vi "analog Variables.vi"(11 "error in (no error)":errorcluster) -> (15 "error out":errorcluster)   [LabVIEW 2011]
uses:
  Variable List Common Digital.ctl
  Fixed Digital Channel Definition.ctl
  Update frequensies.ctl
  Channel catagory Enum.ctl
  <vilib>/Utility/VariantDataType/GetNumericInfo.vi
  emi Lib/Basic/0 - General/App/emi_Application Folder.vi
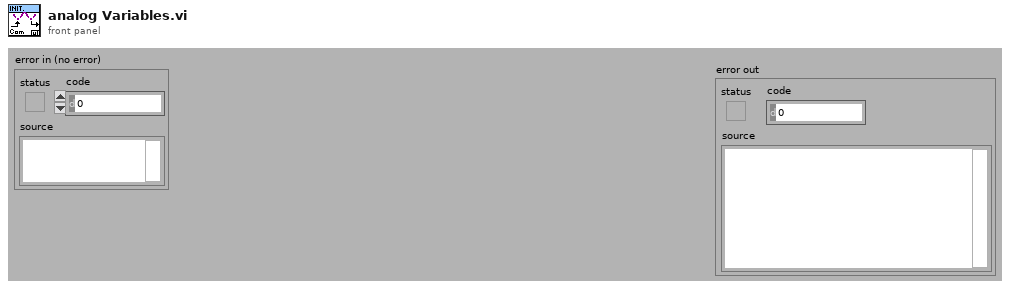
[diagram p1: front panel]
types:
  T1 = typedef "Channel catagory Enum.ctl" = enum16{"No Category", "Power", "Temperature", "Pressure"}
  T2 = typedef "Fixed Digital Channel Definition.ctl" = cluster{"ID":u16, "Name":string, "NA Text":string, "Off Text":string, "On Text":string, "Maximum upd":T3, "Comment":string, "Help file Name":string, "Help file Section ":string, "Catagory":T1, "In use":bool}
  T3 = typedef "Update frequensies.ctl" = enum16{"2 Hz", "1 Hz", "0.1 Hz"}
  T4 = typedef "Variable List Common Digital.ctl" = enum16{"PCP Connected", "PCP PC Control", "HV PSU connected", "HV PSU HV Active", "Modem Connected", "Tool Connected", "CanBus interface"}
  T5 = typedef "Fixed Analog Channel Definition.ctl" = cluster{"ID":u16, "Name":string, "Quantity":T6, "Unit":string, "Maximum upd":T3, "Comment":string, "Help file Name":string, "Help file Section ":string, "Category":T1, "User adjustable Scaling":bool, "Default Scaling":T7, "Default Unit":i32, "Classification":T8}
  T6 = typedef "Quantity enum.ctl" = enum16{"NA", "Acceleration", "Angle", "Current", "Force", "Distance", "Pressure", "Resistance", "Rotational Speed", "Speed", "Temperature", "Tension", "Torque", "Voltage", "Weight"}
  T7 = typedef "Scaling.ctl" = cluster{"Gain":dbl, "Offset":dbl}
  T8 = typedef "Channel Classification Enum.ctl" = enum16{"Basic", "Advanced", "Expert", "Unused"}
  T9 = typedef "User Setting DigitalChannel.ctl" = cluster{"Responses":cluster{"Technical Error (NA)":T10, "OFF / FALSE":T12, "ON / TRUE":T12}}
  T10 = typedef "Alarm Responce.ctl" = cluster{"Action":T11, "Alarm":bool}
  T11 = typedef "Action List.ctl" = enum16{"No Action", "Stop Motor", "Turn Off HV"}
  T12 = typedef "Alarm Responce dig.ctl" = cluster{"Action":T11, "Alarm":bool, "Exclamation":bool}
  T13 = typedef "User Setting Analog Channel Bg.ctl" = cluster{"Scaling":T7, "Limits and responces":T14, "Allow Graph selection by user":bool, "Unit":u16}
  T14 = typedef "Alarm Setup Analog.ctl" = cluster{"Technical Error(NA)":T10, "LL":T10, "L":T10, "H":T10, "HH":T10, "Limits":T15}
  T15 = typedef "Limits.ctl" = cluster{"LL":dbl, "L":dbl, "H":dbl, "HH":dbl}
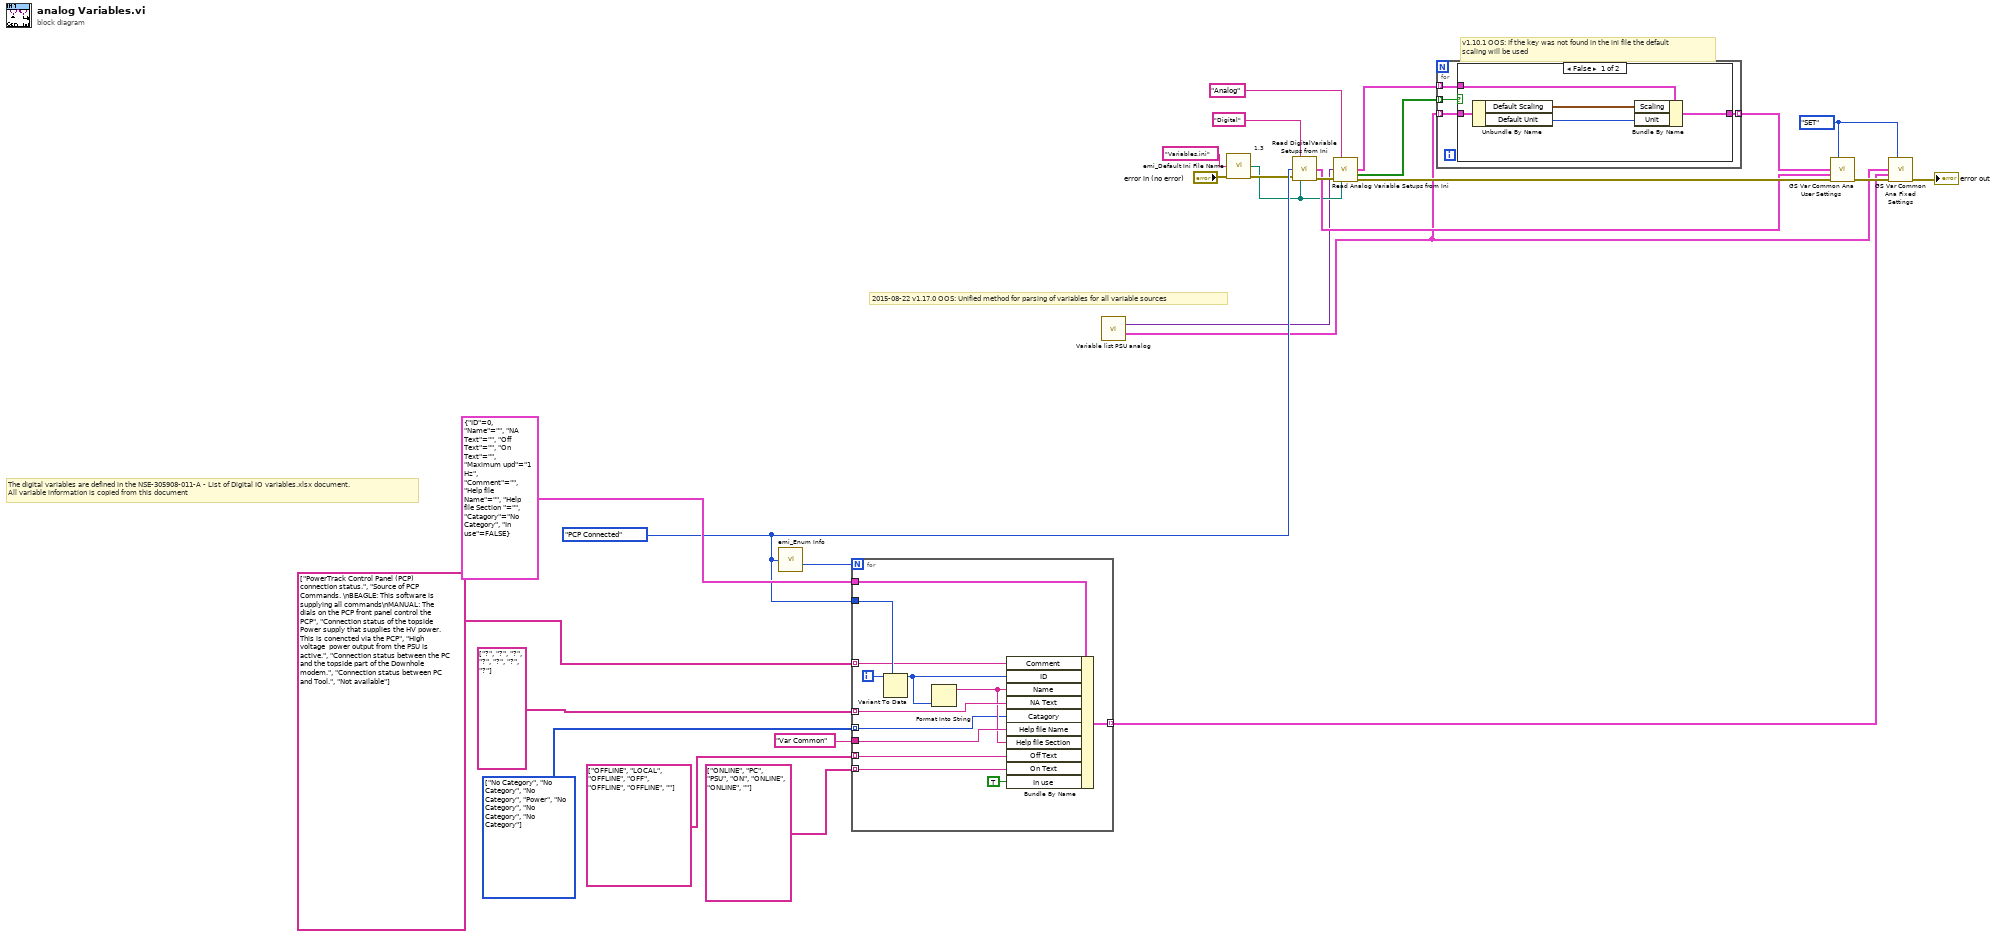
[diagram p0: block diagram]
diagram:
  w18 = T1[] [enum."No Category", enum."No Category", enum."No Category", enum."Power", enum."No Category", enum."No Category", enum."No Category"] items=["No Category", "Power", "Temperature", "Pressure"]
  w12 = Variable_List_Common_Digital."PCP Connected" ("Action")
  w24 = enum16{"GET", "SET"}."SET" ("Action(GET)")
  # "2015-08-22 v1.17.0 OOS: Unified method for parsing of variables for all variable sources"
  # "The digital variables are defined in the NSE-305908-011-A - List of Digital IO variables.xlsx document.\nAll variable information is copied from this document"
  # "v1.10.1 OOS: If the key was not found in the ini file the default\nscaling will be used"
  # "1.3"
  n1 = call "emi_Enum Info.vi"("Enum"=w12) -> ("Numb Elements"=w21:i32)  [unwired: 11 in, 3 out]
  n2 = for {
    N: w21 -> [_]
    tunnel: w12 -> [w40]
    tunnel: T2 {"ID"=0, "Name"="", "NA Text"="", "Off Text"="", "On Text"="", "Maximum upd"=enum."1 Hz", "Comment"="", "Help file Name"="", "Help file Section "="", "Catagory"=enum."No Category", "In use"=FALSE} ("Variable Defenition") -> [w37]
    tunnel: [w38] -> w15 mode=indexing
    tunnel: string[] ["?", "?", "?", "?", "?", "?", "?"] -> [w36] mode=indexing
    tunnel: w18 -> [w32] mode=indexing
    tunnel: "Var Common" -> [w34]
    tunnel: string[] ["OFFLINE", "LOCAL", "OFFLINE", "OFF", "OFFLINE", "OFFLINE", ""] -> [w31] mode=indexing
    tunnel: string[] ["ONLINE", "PC", "PSU", "ON", "ONLINE", "ONLINE", ""] -> [w30] mode=indexing
    tunnel: string[] ["PowerTrack Control Panel (PCP) connection status.", "Source of PCP Commands. \nBEAGLE: This software is supplying all commands\nMANUAL: The dials on the PCP front panel control the PCP", "Connection status of the topside Power supply that supplies the HV power. This is conencted via the PCP", "High voltage  power output from the PSU is active.", "Connection status between the PC and the topside part of the Downhole modem.", "Connection status between PC and Tool.", "Not available"] -> [w29] mode=indexing
    i -> [w35]
    n3 = Variant To Data(type=w40, Variant=w35) -> (data=w39:T4)  [unwired: 1 in, 1 out]
    n4 = Format Into String(w39) -> (resulting string=w33:string)  [unwired: 3 in, 1 out]
    n5 = Bundle By Name(cluster=w37, "Comment"=w29, "ID"=w39, "Name"=w33, "NA Text"=w36, "Catagory"=w32, "Help file Name"=w34, "Help file Section"=w33, "Off Text"=w31, "On Text"=w30, "In use"=TRUE) -> (w38:T2)
  }
  n6 = call "Variable list PSU analog.vi"() -> ("Variant"=w1:variant, "Array"=w2:T5[])  [unwired: 14 in]
  n7 = call "emi_Default Ini File Name.vi"("Name"="Variables.ini" ("name or relative path"), "error in (no error)"="error in (no error)") -> ("Path"=w6:path, "error out"=w8:errorcluster)  [unwired: 12 in]
  n8 = call "Read DigitalVariable Setups from Ini.vi"("error in (no error)"=w8, "Path"=w6, "Enum with Variable List"=w12, "Section(\"Default\")"="Digital" ("Section(\"Default\")")) -> ("error out"=w14:errorcluster, "Digitale User settigns"=w11:T9[])  [unwired: 10 in]
  n9 = call "Read Analog Variable Setups from Ini.vi"("error in (no error)"=w14, "Path"=w6, "Enum with Variable List"=w1, "Section(\"Default\")"="Analog" ("Section(\"Default\")")) -> ("error out"=w27:errorcluster, "Found out"=w4:bool[], "Analog User settigns"=w5:T13[])  [unwired: 9 in]
  n10 = for {
    tunnel: w5 -> [w43] mode=indexing
    tunnel: w4 -> [w44] mode=indexing
    tunnel: w2 -> [w42] mode=indexing
    tunnel: [w41] -> w3 mode=indexing
    n11 = case shown="False" w44 {
      tunnel: w43 -> [w49 w50]
      tunnel: w42 -> [w48 _]
      tunnel: [w45 w50] -> w41
      frame False {
        n12 = Unbundle By Name(w48) -> ("Default Scaling"=w47:T7, "Default Unit"=w46:i32)
        n13 = Bundle By Name(cluster=w49, "Scaling"=w47, "Unit"=w46) -> (w45:T13)
      }
      frame True {
      }
    }
  }
  n14 = call "GS Var Common Ana User Settings.vi"("Action(GET)"=w24, "Common variables User settigns in"=w3, "Common Digital Var User set in"=w11, "error in (no error)"=w27) -> ("error out"=w26:errorcluster)  [unwired: 9 in, 2 out]
  n15 = call "GS Var Common Ana Fixed Settings.vi"("Action(GET)"=w24, "Common Analog Var Fixed in"=w2, "Common Digital Var Fixed in"=w15, "error in (no error)"=w26) -> ("error out"=→"error out":errorcluster)  [unwired: 9 in, 2 out]
